vi "TestPFGVPersonnelManagment.vi"() -> (0 "error out":errorcluster, 2 "Pass":bool)   [LabVIEW 2015]
uses:
  TypeDef/PersonnelActions.ctl
  LVClasses/Personnel/PersonnelType.ctl
  LVClasses/Flags/Flags.lvclass
  LVClasses/Room/Room.lvclass
  LVClasses/Personnel/Personnel.lvclass
panel:
  out "Added":bool
  out "Removed?":bool
  out "DataInit PUIDs":string
  out "Add Personnel 2":string
  out "Read PUIDs 2":string
  out "Remove Personnel":string
  out "Add Personnel":string
  out "Read PUIDS":string
  in  "PUID":string="d1"
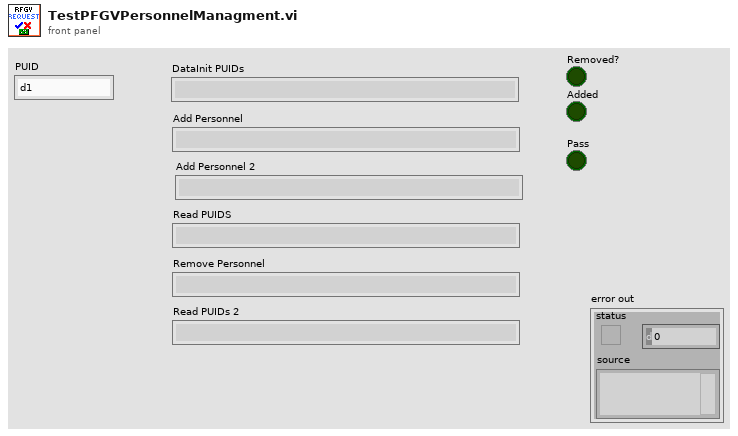
[diagram p1: front panel]
types:
  T1 = typedef "Personnel.lvclass/PersonnelType.ctl" = enum16{"Nurse", "Doctor", "Cleanning", "Admin"}
  T2 = typedef "PersonnelActions.ctl" = enum16{"Init", "Read Personnel", "Add Personnel", "Remove Personnel", "Read Name", "Write Name", "Read Role", "Write Role", "Read Requests", "Add Requests", "Remove Requests", "Read PUIDs"}
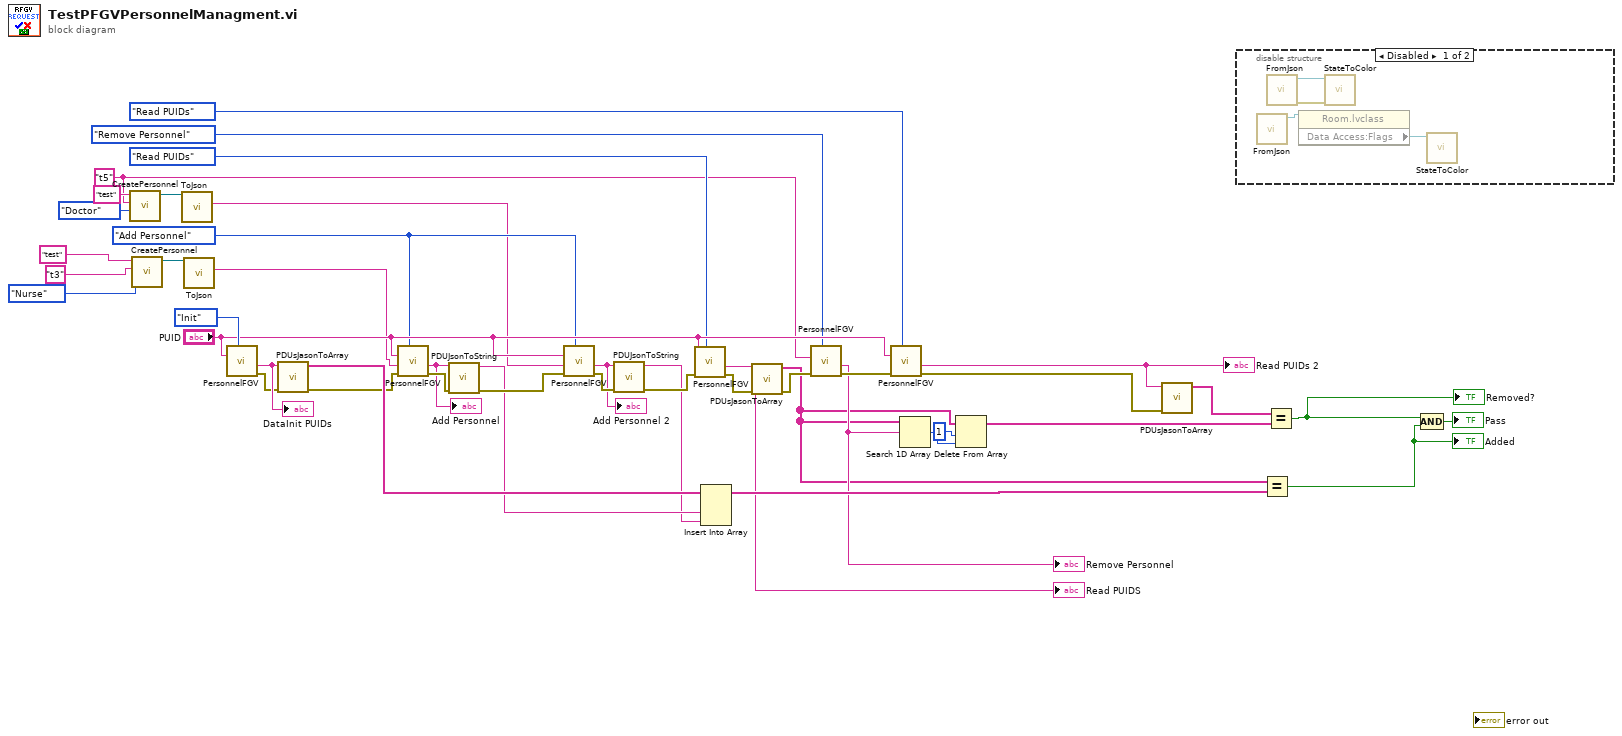
[diagram p0: block diagram]
diagram:
  w1 = "t5" ("UniqueID")
  w36 = PersonnelActions."Add Personnel" ("Actions")
  n1 = call "CreatePersonnel.vi"("Role"=PersonnelType."Doctor", "UniqueID"=w1, "Name"="test") -> ("output cluster"=w35:refnum<class "Personnel.lvclass">)  [unwired: 7 in, 1 out]
  n2 = call "CreatePersonnel.vi"("Role"=PersonnelType."Nurse", "UniqueID"="t3", "Name"="test") -> ("output cluster"=w34:refnum<class "Personnel.lvclass">)  [unwired: 7 in, 1 out]
  n3 = call "ToJson.vi"("Personnel in"=w35) -> ("PersonnelJson"=w2:string)  [unwired: 8 in, 2 out]
  n4 = call "ToJson.vi"("Personnel in"=w34) -> ("PersonnelJson"=w33:string)  [unwired: 8 in, 2 out]
  n5 = call "PersonnelFGV.vi"("Actions"=PersonnelActions."Init", "PUID"="PUID") -> ("error out"=w24:errorcluster, "Data Out"=w27:string)  [unwired: 8 in]
  "DataInit PUIDs" <- w27
  n6 = call "PDUsJasonToArray.vi"("error in (no error)"=w24, "Data Out"=w27) -> ("error out"=w23:errorcluster, "PUIDs"=w25:string[])  [unwired: 8 in]
  n7 = call "PersonnelFGV.vi"("Actions"=w36, "error in (no error)"=w23, "Data In"=w33, "PUID"="PUID") -> ("error out"=w19:errorcluster, "Data Out"=w12:string)  [unwired: 6 in]
  "Add Personnel" <- w12
  n8 = call "PDUJsonToString.vi"("error in (no error)"=w19, "Data Out"=w12) -> ("error out"=w18:errorcluster, "PUID"=w10:string)  [unwired: 8 in]
  n9 = call "PersonnelFGV.vi"("Actions"=w36, "error in (no error)"=w18, "Data In"=w2, "PUID"="PUID") -> ("error out"=w17:errorcluster, "Data Out"=w11:string)  [unwired: 6 in]
  "Add Personnel 2" <- w11
  n10 = call "PDUJsonToString.vi"("error in (no error)"=w17, "Data Out"=w11) -> ("error out"=w16:errorcluster, "PUID"=w9:string)  [unwired: 8 in]
  n11 = call "PersonnelFGV.vi"("Actions"=PersonnelActions."Read PUIDs", "error in (no error)"=w16, "PUID"="PUID") -> ("error out"=w15:errorcluster, "Data Out"=w8:string)  [unwired: 7 in]
  "Read PUIDS" <- w8
  n12 = Insert Into Array(array=w25, new element #1=w10, new element #2=w9) -> (w26:string[])  [unwired: 1 in]
  n13 = call "PDUsJasonToArray.vi"("error in (no error)"=w15, "Data Out"=w8) -> ("error out"=w14:errorcluster, "PUIDs"=w4:string[])  [unwired: 8 in]
  n14 = call "PersonnelFGV.vi"("Actions"=PersonnelActions."Remove Personnel", "error in (no error)"=w14, "PUID"=w1) -> ("error out"=w13:errorcluster, "Data Out"=w7:string)  [unwired: 7 in]
  "Remove Personnel" <- w7
  n15 = call "PersonnelFGV.vi"("Actions"=PersonnelActions."Read PUIDs", "error in (no error)"=w13, "PUID"="PUID") -> ("error out"=w21:errorcluster, "Data Out"=w22:string)  [unwired: 7 in]
  "Read PUIDs 2" <- w22
  n16 = Search 1D Array(1D array=w4, element=w7) -> (index of element=w6:i32)  [unwired: 1 in]
  n17 = Delete From Array(array=w4, length=1, index=w6) -> (array with subset deleted=w3:string[])  [unwired: 1 out]
  n18 = call "PDUsJasonToArray.vi"("error in (no error)"=w21, "Data Out"=w22) -> ("PUIDs"=w20:string[])  [unwired: 8 in, 1 out]
  n19 = disable-structure shown="Disabled" {
    frame Disabled {
      n20 = call "FromJson.vi"() -> ("Room out"=w46:refnum<class "Room.lvclass">)  [unwired: 10 in, 1 out]
      n21 = call "FromJson.vi"() -> ("error out"=w48:errorcluster, "Flags out"=w47:refnum<class "Flags.lvclass">)  [unwired: 10 in]
      n22 = property class="Room.lvclass"(reference=w46) -> ("Data Access:Flags"=w45:refnum<class "Flags.lvclass">)  [unwired: 1 in, 2 out]
      n23 = call "StateToColor.vi"("error in (no error)"=w48, "Flags in"=w47) -> ()  [unwired: 7 in, 3 out]
      n24 = call "StateToColor.vi"("Flags in"=w45) -> ()  [unwired: 8 in, 3 out]
    }
    frame Enabled {
    }
  }
  n25 = Equal?(x=w4, y=w26) -> (x = y?=w42:bool)
  "Added" <- w42
  n26 = Equal?(x=w20, y=w3) -> (x = y?=w44:bool)
  "Removed?" <- w44
  n27 = Compound Arithmetic op=AND(w44, w42) -> (→"Pass":bool)
